vi "Create Log File.vi"(8 "error in":errorcluster, 11 "File Path (use dialog)":path=path "C:/testlog.txt") -> (0 "error out":errorcluster, 3 "log file path":path)   [LabVIEW 2016]
uses:
  <vilib>/Utility/file.llb/Write Delimited Spreadsheet (string).vi
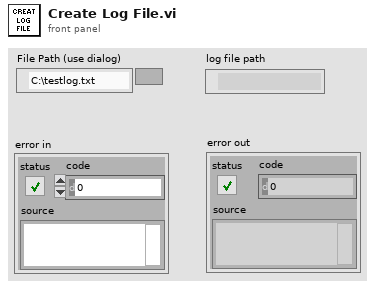
[diagram p1: front panel]
types:
  T1 = enum16{"open", "replace", "create", "open or create", "replace or create", "replace or create with confirmation"}
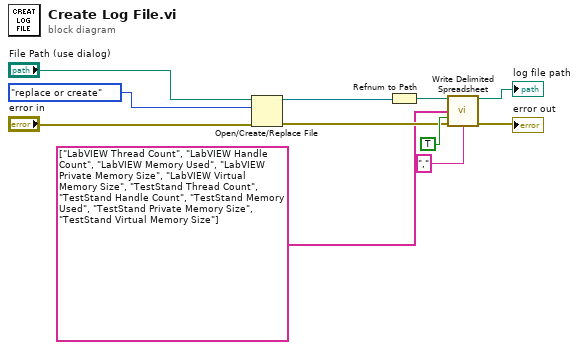
[diagram p0: block diagram]
diagram:
  n1 = Open/Create/Replace File(file path (use dialog)="File Path (use dialog)", error in="error in", operation (0:open)=T1."replace or create") -> (refnum out=w9:refnum<file>, error out=w8:errorcluster)  [unwired: 3 in, 1 out]
  n2 = Refnum to Path(1:w9) -> (0:w10:path)
  n3 = call-poly <vilib>:"Write Delimited Spreadsheet.vi"("file path (dialog if empty)"=w10, "1D data"=string[] ["LabVIEW Thread Count", "LabVIEW Handle Count", "LabVIEW Memory Used", "LabVIEW Private Memory Size", "LabVIEW Virtual Memory Size", "TestStand Thread Count", "TestStand Handle Count", "TestStand Memory Used", "TestStand Private Memory Size", "TestStand Virtual Memory Size"], "append to file? (new file:F)"=TRUE, "error in (no error)"=w8, "delimiter (\\t)"="," ("delimiter (\\t)")) -> ("new file path (Not A Path if cancelled)"=→"log file path":path, "error out"=→"error out":errorcluster)  [unwired: 9 in]
